vi "SetHomeOffset.vi"(8 "Error In":errorcluster, 10 "Offset":dbl, 11 "Thorlabs In":refnum<class "Thorlabs.lvclass">) -> (0 "Error Out":errorcluster, 3 "Thorlabs Out":refnum<class "Thorlabs.lvclass">)   [LabVIEW 2018, in "Thorlabs.lvlib" / "Thorlabs.lvclass"]
doc: "This VI sets the offset for the Home command.\n\nCreator: Slade Jeppesen\nCreated Date: 09/29/20"
uses:
  Thorlabs.lvclass
  Thorlabs.lvclass/Thorlabs.ctl
  C:/AME Test Engineering/LabVIEW/PPLs/Axis/DLLs/ThorLabs.MotionControl.KCube.DCServoCLI.dll
  PPLs/Axis/DLLs/ThorLabs.MotionControl.KCube.DCServoCLI.dll
  C:/AME Test Engineering/LabVIEW/PPLs/Axis/DLLs/Thorlabs.MotionControl.GenericMotorCLI.dll
  PPLs/Axis/DLLs/Thorlabs.MotionControl.GenericMotorCLI.dll
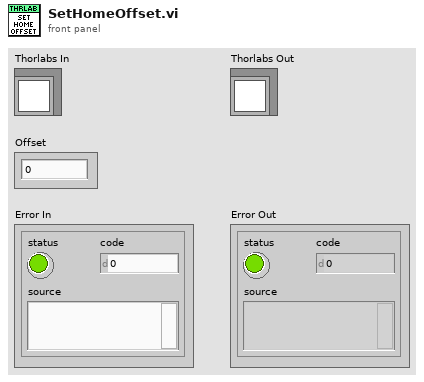
[diagram p1: front panel]
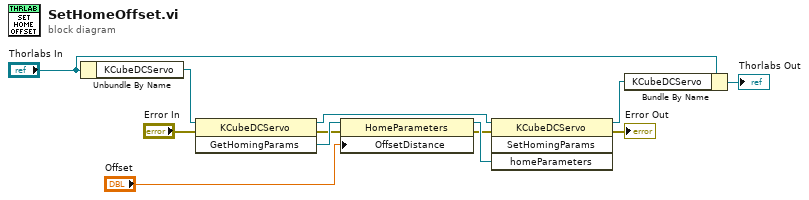
[diagram p0: block diagram]
diagram:
  n1 = Unbundle By Name("Thorlabs In") -> ("KCubeDCServo"=w12:refnum<k24>)
  n2 = invoke class="KCubeDCServo" method="GetHomingParams"(reference=w12, error in="Error In") -> (reference out=w9:refnum<k24>, error out=w5:errorcluster, "GetHomingParams"=w11:refnum<k24>)  [unwired: 1 in]
  n3 = property class="HomeParameters"(reference=w11, error in=w5, "OffsetDistance"="Offset") -> (reference out=w10:refnum<k24>, error out=w4:errorcluster)
  n4 = invoke class="KCubeDCServo" method="SetHomingParams"(reference=w9, error in=w4, "homeParameters"=w10) -> (reference out=w8:refnum<k24>, error out=→"Error Out":errorcluster)  [unwired: 1 in, 2 out]
  n5 = Bundle By Name(cluster="Thorlabs In", "KCubeDCServo"=w8) -> (→"Thorlabs Out":refnum<class "Thorlabs.lvclass">)
